vi "Run Execution Loop Start Callbacks.vi"(8 "error in (no error)":errorcluster, 11 "Execution in":refnum<data-value>) -> (0 "error out":errorcluster, 3 "Execution out":refnum<data-value>)   [LabVIEW 2015, in "Execution.lvclass"]
uses:
  Execution.lvclass
  Project.lvclass
  Plugin.lvclass
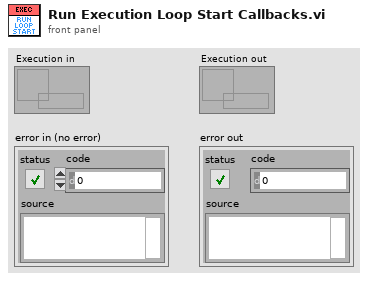
[diagram p1: front panel]
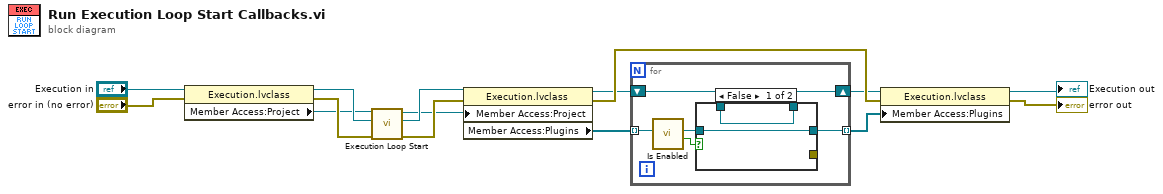
[diagram p0: block diagram]
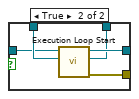
[diagram p2: hidden frame]
diagram:
  n1 = property class="Execution.lvclass"(reference="Execution in", error in="error in (no error)") -> (reference out=w14:refnum<data-value>, error out=w2:errorcluster, "Member Access:Project"=w1:refnum<class "Project.lvclass">)
  n2 = call-dynamic "Execution Loop Start.vi"("error in (no error)"=w2, "Execution in"=w14, "Project in"=w1) -> ("error out"=w4:errorcluster, "Execution out"=w15:refnum<data-value>, "Project out"=w3:refnum<class "Project.lvclass">)  [unwired: 6 in]
  n3 = property class="Execution.lvclass"(reference=w15, error in=w4, "Member Access:Project"=w3) -> (reference out=w7:refnum<data-value>, error out=w11:errorcluster, "Member Access:Plugins"=w8:refnum<class "Plugin.lvclass">[])
  n4 = for {
    tunnel: w8 -> [w18] mode=indexing
    shift-right: [w19] -> w9
    shift-left: w7 -> [w20]
    tunnel: [w21] -> w10 mode=indexing
    n5 = call "Is Enabled.vi"("Plugin in"=w18) -> ("Enabled"=w16:bool, "Plugin out"=w17:refnum<class "Plugin.lvclass">)  [unwired: 9 in]
    n6 = case shown="False" w16 {
      tunnel: [w22 w28] -> w21
      tunnel: [_ w27] -> _
      tunnel: w20 -> [w23 w26]
      tunnel: [w23 w25] -> w19
      tunnel: w17 -> [w22 w24]
      frame False {
      }
      frame True {
        n7 = call-dynamic "Execution Loop Start.vi"("Execution in"=w26, "Plugin in"=w24) -> ("error out"=w27:errorcluster, "Execution out"=w25:refnum<data-value>, "Plugin out"=w28:refnum<class "Plugin.lvclass">)  [unwired: 7 in]
      }
    }
  }
  n8 = property class="Execution.lvclass"(reference=w9, error in=w11, "Member Access:Plugins"=w10) -> (reference out=→"Execution out":refnum<data-value>, error out=→"error out":errorcluster)
